vi "Get AIO Info.vi"(8 "Error In":errorcluster, 11 "LINX Resource":T2={"IO"=enum."Remote", "Interface"=enum."Serial", "LINX Device Config"={"Interface"=enum."Serial", "COM Port"="COM13", "TCP Configuration"={"IP Address"="", "Port"=0}, "Device Family"=1, "Device ID"=1, "Device Name"="myRIO-1900", "TCP Ref"=refnum, "Channels"={"DI"=[0, 1, 2, 3, 4, 5, 6, 7, 8, 9, 10, 11, 12, 13, 14, 15, 16, 17, 18, 19, 20, 21, 22, 23, 24, 25, 26, 27, 28, 29, 30, 31, 32, 33, 34, 35, 36, 37, 38, 39, 40, 41, 42, 43, 44, 45, 46], "DO"=[0, 1, 2, 3, 4, 5, 6, 7, 8, 9, 10, 11, 12, 13, 14, 15, 16, 17, 18, 19, 20, 21, 22, 23, 24, 25, 26, 27, 28, 29, 30, 31, 32, 33, 34, 35, 36, 37, 38, 39, 40, 41, 42, 43, 44, 45, 46], "AI"=[0, 1, 2, 3, 4, 5, 6, 7, 8, 9, 10, 11], "AO"=[], "PWM"=[3, 5, 6, 9, 10], "QE"=[], "UART"=[0, 1], "I2C 2"=[0], "SPI"=[0], "CAN"=[], "Servo"=[], "AI Ref (V)"=0.0, "AI Resolution (Bits)"=0, "AO Ref (V)"=0.0, "AO Resolution (Bits)"=0}}}) -> (0 "Error Out":errorcluster, 1 "AO info":T1, 2 "AI info":T1, 3 "LINX resource":T2)   [LabVIEW 2019, in "LINXx.lvlib"]
doc: "Gets analog input & output capability info from LINX board"
uses:
  LINXx.lvlib
  <vilib>/MakerHub/LINX/Private/Type Defs/LINX Ref.ctl
  <vilib>/MakerHub/LINX/Private/Type Defs/Platform.ctl
  <vilib>/MakerHub/LINX/Private/Type Defs/Interface.ctl
  <vilib>/MakerHub/LINX/Private/Device/Type Defs/LINX Device Config.ctl
  <vilib>/MakerHub/LINX/Private/Device/Type Defs/TCP Config.ctl
  <vilib>/MakerHub/LINX/Private/Device/Type Defs/Channels.ctl
  Private/Analog info.ctl
  <vilib>/MakerHub/LINX/LMH-LINX.lvlib
  <vilib>/MakerHub/LINX/Private/Device/Device.lvlib
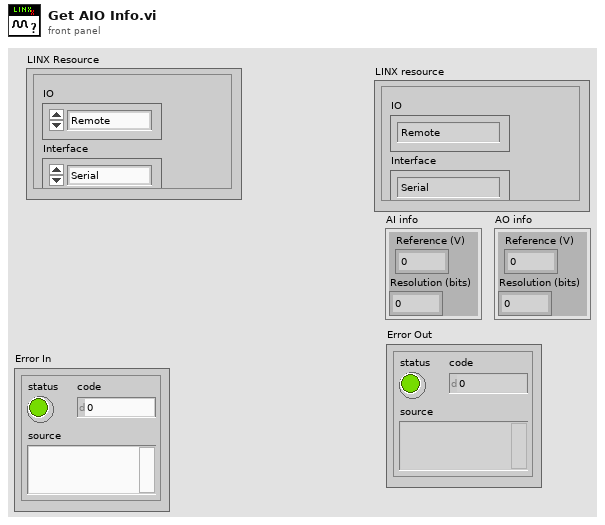
[diagram p1: front panel]
types:
  T1 = typedef "LINXx.lvlib/Analog info.ctl" = cluster{"Reference (V)":dbl, "Resolution (bits)":u8}
  T2 = typedef "LMH-LINX.lvlib/LINX Ref.ctl" = cluster{"IO":T3, "Interface":T4, "LINX Device Config":T5}
  T3 = typedef "LMH-LINX.lvlib/Platform.ctl" = enum16{"Remote", "Local"}
  T4 = typedef "LMH-LINX.lvlib/Interface.ctl" = enum16{"Serial", "TCP"}
  T5 = typedef "LMH-LINX.lvlib/Device.lvlib/LINX Device Config.ctl" = cluster{"Interface":T4, "COM Port":refnum<visa-resource-name>, "TCP Configuration":T6, "Device Family":u8, "Device ID":u8, "Device Name":string, "TCP Ref":refnum<k5>, "Channels":T7}
  T6 = typedef "LMH-LINX.lvlib/Device.lvlib/TCP Config.ctl" = cluster{"IP Address":string, "Port":u16}
  T7 = typedef "LMH-LINX.lvlib/Channels.ctl" = cluster{"DI":u8[], "DO":u8[], "AI":u8[], "AO":u8[], "PWM":u8[], "QE":u8[], "UART":u8[], "I2C 2":u8[], "SPI":u8[], "CAN":u8[], "Servo":u8[], "AI Ref (V)":dbl, "AI Resolution (Bits)":u8, "AO Ref (V)":dbl, "AO Resolution (Bits)":u8}
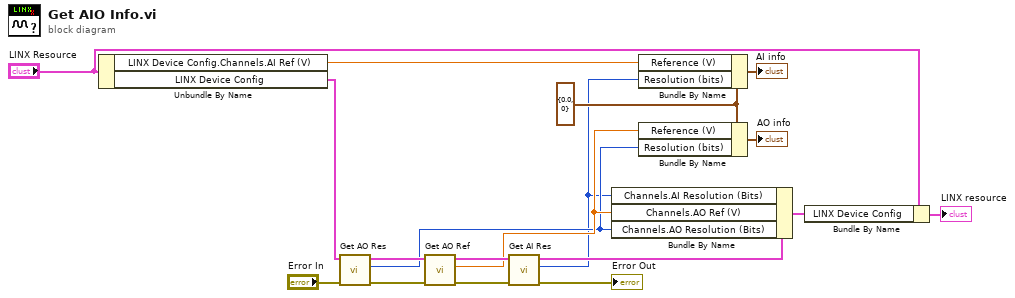
[diagram p0: block diagram]
diagram:
  w7 = T1 {"Reference (V)"=0.0, "Resolution (bits)"=0} ("Analog info")
  n1 = Unbundle By Name("LINX Resource") -> ("LINX Device Config.Channels.AI Ref (V)"=w3:dbl, "LINX Device Config"=w9:T5)
  n2 = call "Get AO Res.vi"("Error In"="Error In", "LINX Device Config"=w9) -> ("Error Out"=w12:errorcluster, "AO Res"=w5:u8, "LINX Device Config"=w15:T5)  [unwired: 7 in]
  n3 = call "Get AO Ref.vi"("Error In"=w12, "LINX Device Config"=w15) -> ("Error Out"=w13:errorcluster, "AO Ref"=w6:dbl, "LINX Device Config"=w14:T5)  [unwired: 7 in]
  n4 = call "Get AI Res.vi"("Error In"=w13, "LINX Device Config"=w14) -> ("Error Out"=→"Error Out":errorcluster, "AI Res"=w4:u8, "LINX Device Config"=w18:T5)  [unwired: 7 in]
  n5 = Bundle By Name(cluster=w18, "Channels.AI Resolution (Bits)"=w4, "Channels.AO Ref (V)"=w6, "Channels.AO Resolution (Bits)"=w5) -> (w10:T5)
  n6 = Bundle By Name(cluster=w7, "Reference (V)"=w3, "Resolution (bits)"=w4) -> (→"AI info":T1)
  n7 = Bundle By Name(cluster=w7, "Reference (V)"=w6, "Resolution (bits)"=w5) -> (→"AO info":T1)
  n8 = Bundle By Name(cluster="LINX Resource", "LINX Device Config"=w10) -> (→"LINX resource":T2)
